vi "Write Case sensitive.vi"(5 "Case sensitive":bool, 9 "Combobox in":refnum<class "Combobox.lvclass">) -> (3 "Combobox out":refnum<class "Combobox.lvclass">)   [LabVIEW 2014, in "Combobox.lvclass"]
uses:
  Combobox.lvclass
  Combobox.lvclass/Combobox.ctl
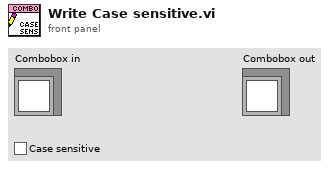
[diagram p1: front panel]
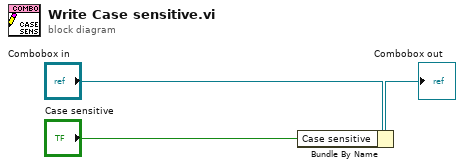
[diagram p0: block diagram]
diagram:
  n1 = Bundle By Name(cluster="Combobox in", "Case sensitive"="Case sensitive") -> (→"Combobox out":refnum<class "Combobox.lvclass">)
